vi "LS 340 get T.vi"(0 "GPIB Adress":i16) -> (3 "Temperature":dbl format="%.3f")   [LabVIEW 2015]
panel:
  in  "error in (no error)":errorcluster
  out "error out":errorcluster
  out "data string":string
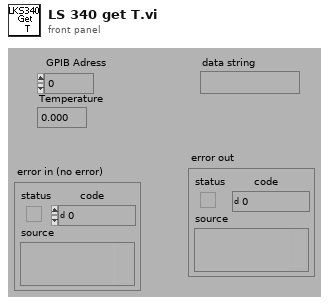
[diagram p1: front panel]
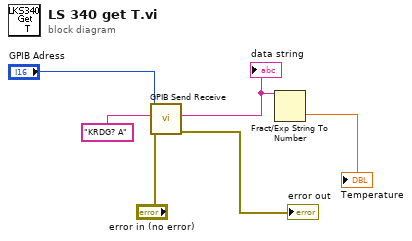
[diagram p0: block diagram]
diagram:
  n1 = call "GPIB Send Receive.vi"("error in (no error)"="error in (no error)", "data string in"="KRDG? A" ("data string"), "GPIB Adress"="GPIB Adress") -> ("error out"=→"error out":errorcluster, "data string out"=w3:string)  [unwired: 6 in, 1 out]
  "data string" <- w3
  n2 = Fract/Exp String To Number(string=w3) -> (number=→"Temperature":dbl)  [unwired: 3 in, 1 out]
